vi "Core_Module.vi"() -> ()   [LabVIEW 2023]
uses:
  <vilib>/regexp/Match Regular Expression.xnode
panel:
  out "Error_Out":errorcluster
  in  "Error_In":errorcluster
  in  "Wait_Time (sec)":i32
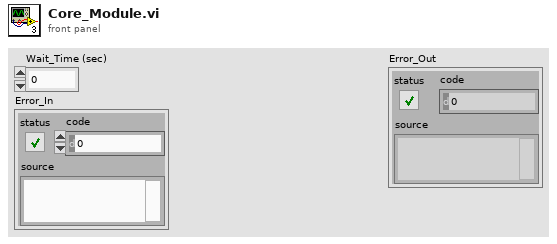
[diagram p1: front panel]
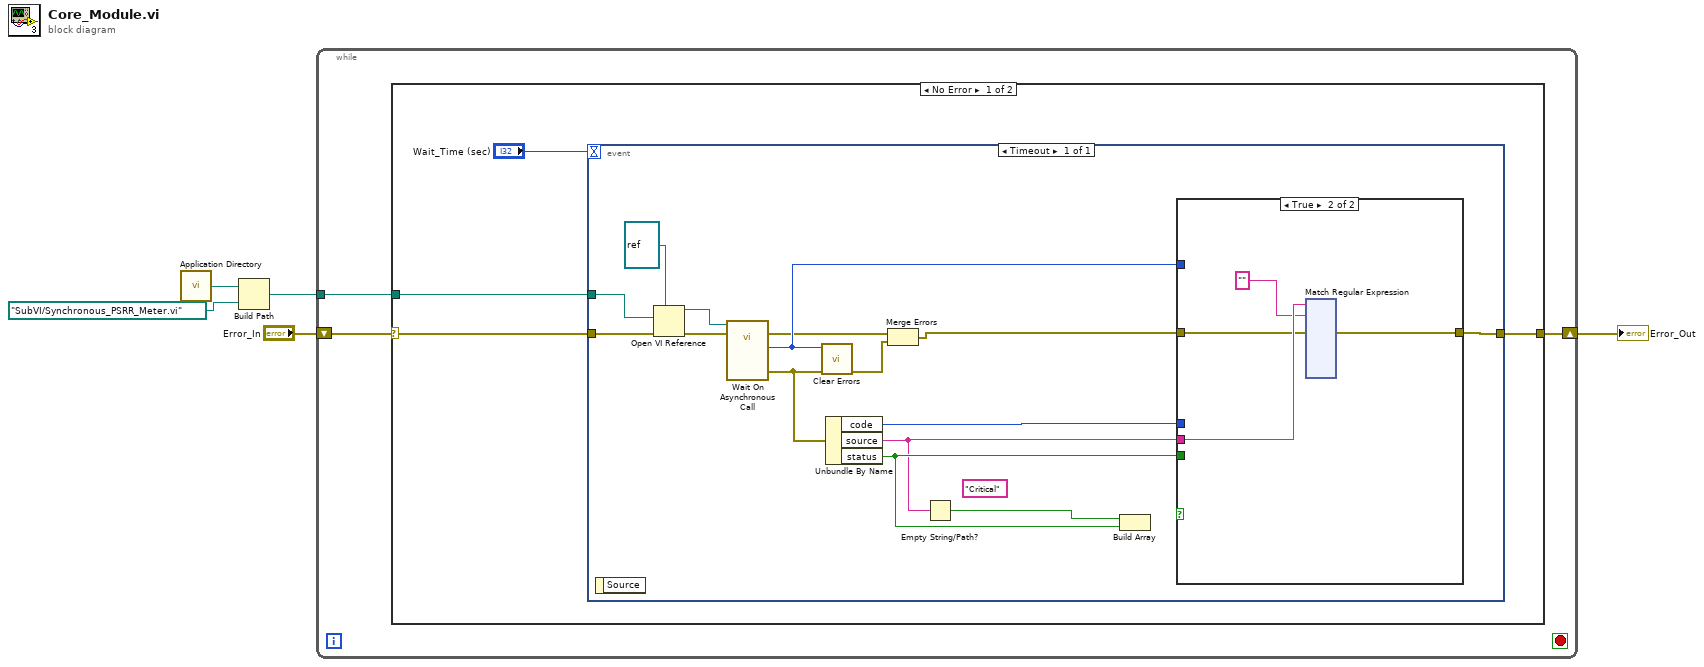
[diagram p0: block diagram]
diagram:
  n1 = call <vilib>:"Application Directory.vi"() -> ("Application Directory"=w3:path)
  n2 = Build Path(base path=w3, name or relative path=path "SubVI/Synchronous_PSRR_Meter.vi") -> (appended path=w1:path)
  n3 = while {
    shift-right: [w6] -> w4
    shift-left: "Error_In" -> [w8]
    tunnel: w1 -> [w7]
    stop <- _ stop-if-true
    n4 = case shown="No Error" w8 {
      selector: w8 -> [w10 _]
      tunnel: w7 -> [w11 _]
      tunnel: [w9 _] -> w6
      frame No Error {
        n5 = event shown="[0] Timeout" {
          selector: _ -> [_]
          dyn-events: _ -> [_]
          timeout: "Wait_Time (sec)" -> [_]
          tunnel: w11 -> [w25]
          tunnel: w10 -> [w18]
          tunnel: [w16] -> w9
          event Timeout {
            (unwired) "Critical" ("true string")
            n6 = event-data() -> ()  [unwired: 1 in, 1 out]
            n7 = Open VI Reference(type specifier VI Refnum (for type only)=refnum<vi> refnum, vi path=w25, error in (no error)=w18) -> (vi reference=w27:refnum<vi>, error out=w17:errorcluster)  [unwired: 3 in]
            n8 = call-by-ref "Wait On Asynchronous Call"(reference=w27, error in=w17) -> (error out=w15:errorcluster, 0:"error out"=w20:errorcluster, "PSRR (dB)"=w19:i32)  [unwired: 10 in, 1 out]
            n9 = call <vilib>:"Clear Errors.vi"("error in (no error)"=w20, "specific error code to clear (0: all)"=w19) -> ("error out"=w13:errorcluster)  [unwired: 4 in, 1 out]
            n10 = Unbundle By Name(w20) -> ("code"=w23:i32, "source"=w21:string, "status"=w24:bool)
            n11 = Merge Errors(w15, w13) -> (w14:errorcluster)
            n12 = Empty String/Path?(string/path=w21) -> (empty?=w22:bool)
            n13 = Build Array(w22, w24) -> ()  [unwired: 1 out]
            n14 = case shown="True" {
              selector: _ -> [_ _]
              tunnel: w21 -> [_ w31]
              tunnel: w24 -> [_ _]
              tunnel: w19 -> [_ _]
              tunnel: w23 -> [_ _]
              tunnel: w14 -> [_ w29]
              tunnel: [_ w28] -> w16
              frame False {
              }
              frame True {
                n15 = xnode "Match Regular Expression"("input string"=w31, "regular expression"="", "error in"=w29) -> ("error out"=w28:errorcluster)  [unwired: 3 in, 9 out]
              }
            }
          }
        }
      }
      frame Error {
      }
    }
  }
  "Error_Out" <- w4
